vi "Tach Process Analog (1 Ch).vi"(0 "analog tacho signal":sgl[](array[numeric]), 1 "sampling rate [Hz]":dbl=1.0, 2 "threshold":dbl format="%.2f", 3 "pulse/revolution (1)":i32=1, 4 "slope (Rising)":u16(ring) items=["Rising", "Falling"], 5 "hysteresis (0)":dbl format="%.2f", 7 "pulse width (2)":i32=2, 8 "Empty Block Cutoff":i32, 9 "tach state in":T1) -> (13 "tach state out":T1, 14 "speed position info":T3, 15 "binary tach signal":sgl[](array[numeric]), 18 "Instant RPM":dbl)   [LabVIEW 2017, in "VibrationAnalysisFunctions.lvlib"]
uses:
  <vilib>/addons/InsightCM/Utilities/Analysis/Vibration/VibrationAnalysisFunctions.lvlib
  <vilib>/addons/Sound and Vibration/Order Analysis/Misc/OAT Position Info.ctl
  <vilib>/addons/InsightCM/Utilities/Analysis/Vibration/controls/Tachometer.ctl
  <vilib>/addons/InsightCM/Utilities/Analysis/Vibration/controls/DigitalTachometer.ctl
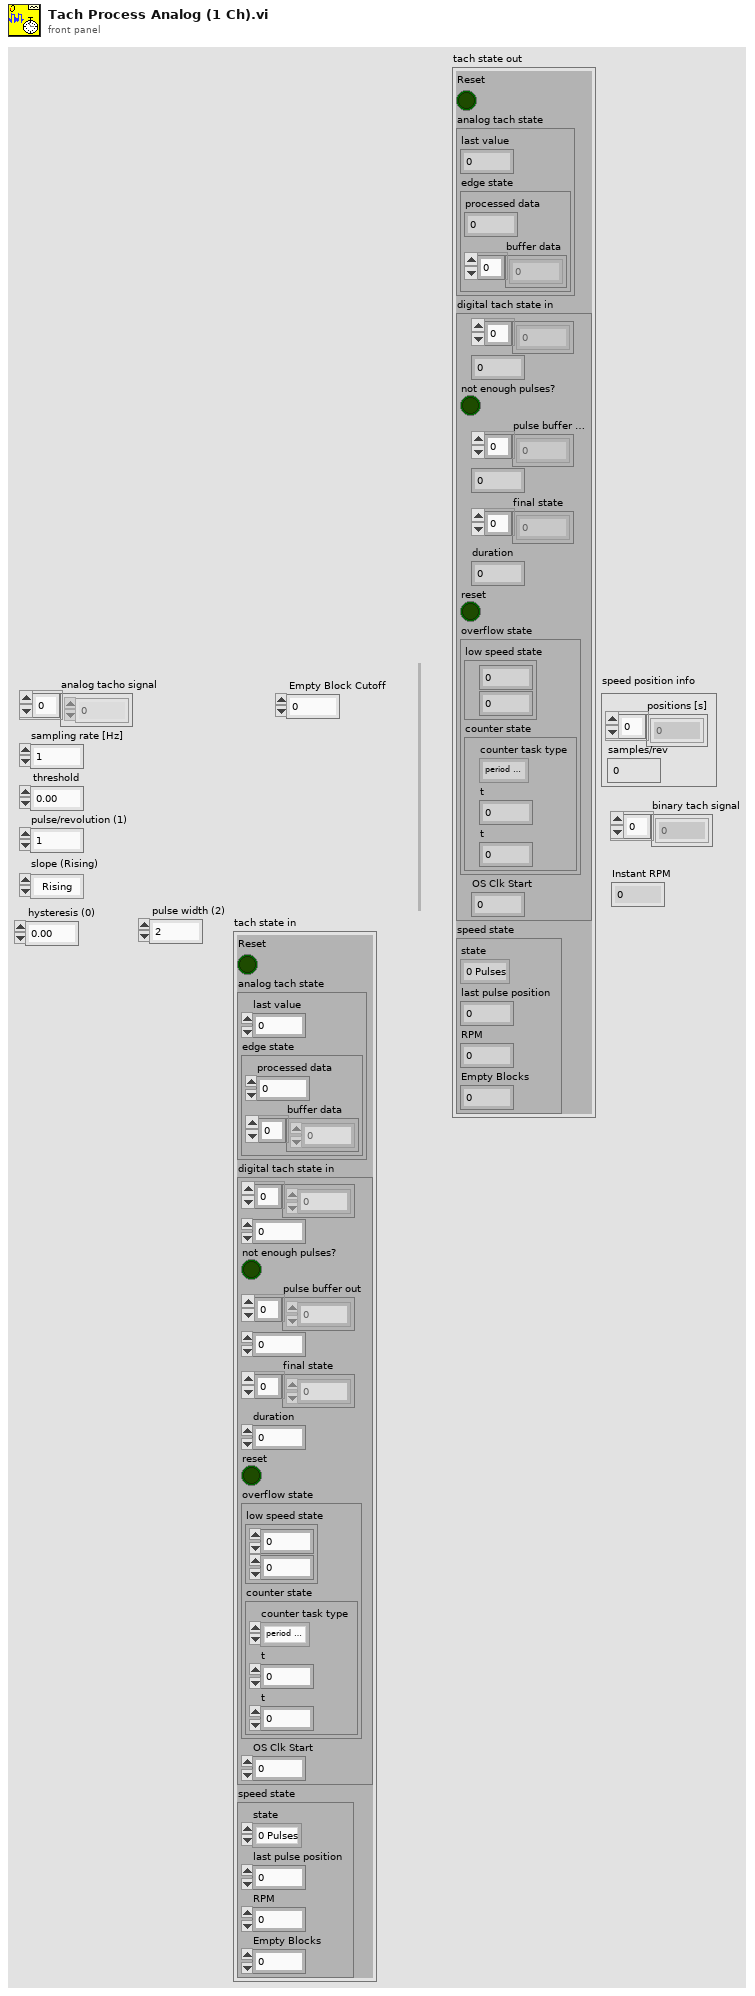
[diagram p1: front panel]
types:
  T1 = typedef "VibrationAnalysisFunctions.lvlib/Tachometer.ctl" = cluster{"Reset":bool, "analog tach state":cluster{"last value":dbl, "edge state":cluster{"processed data":dbl, "buffer data":dbl[]}}, "digital tach state in":T2, "speed state":cluster{"state":enum16{"0 Pulses", "1 Pulse", "2+ Pulses"}, "last pulse position":dbl, "RPM":dbl, "Empty Blocks":i32}}
  T2 = typedef "VibrationAnalysisFunctions.lvlib/DigitalTachometer.ctl" = cluster{dbl[], i32, "not enough pulses?":bool, "pulse buffer out":dbl[], i32, "final state":dbl[], "duration":dbl, "reset":bool, "overflow state":cluster{"low speed state":cluster{dbl, ext}, "counter state":cluster{"counter task type":enum16{"period measurement", "event counting"}, "t":dbl, "t":dbl}}, "OS Clk Start":dbl}
  T3 = typedef "OAT Position Info.ctl" = cluster{"positions [s]":dbl[], "samples/rev":dbl}
  T4 = cluster{"last value":dbl, "edge state":cluster{"processed data":dbl, "buffer data":dbl[]}}
  T5 = cluster{"state":enum16{"0 Pulses", "1 Pulse", "2+ Pulses"}, "last pulse position":dbl, "RPM":dbl, "Empty Blocks":i32}
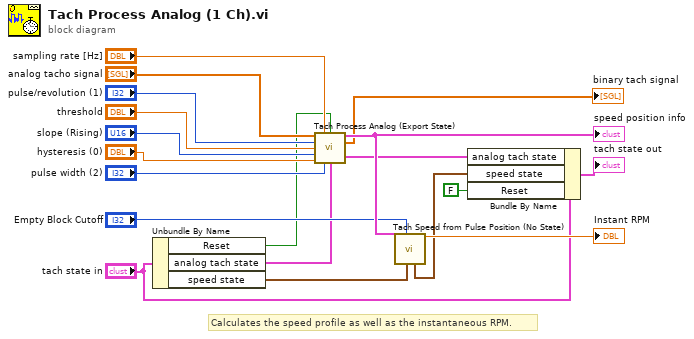
[diagram p0: block diagram]
diagram:
  # "Calculates the speed profile as well as the instantaneous RPM."
  n1 = Unbundle By Name("tach state in") -> ("Reset"=w2:bool, "analog tach state"=w7:T4, "speed state"=w8:T5)
  n2 = call <vilib>:"Tach Process Analog (Export State).vi"("input signal"="analog tacho signal", "sampling rate [Hz]"="sampling rate [Hz]", "reset? (F)"=w2, "PPR"="pulse/revolution (1)", "Thresh(V)"="threshold", "Slope"="slope (Rising)", "hysteresis (0)"="hysteresis (0)", "pulse width (2)"="pulse width (2)", "state in"=w7) -> ("speed position info"=w15:T3, "binary tach signal"=→"binary tach signal":sgl[], "state out"=w11:T4)  [unwired: 4 in]
  "speed position info" <- w15
  n3 = call <vilib>:"Tach Speed from Pulse Position (No State).vi"("state in"=w8, "Empty Block Cutoff"="Empty Block Cutoff", "speed position info"=w15) -> ("RPM"=→"Instant RPM":dbl, "state out"=w10:T5)  [unwired: 7 in]
  n4 = Bundle By Name(cluster="tach state in", "analog tach state"=w11, "speed state"=w10, "Reset"=FALSE) -> (→"tach state out":T1)
